vi "CookieGameEngine.vi"() -> (0 "PlayAgain":bool)   [LabVIEW 2020]
uses:
  typeDef/StateMachineEnum.ctl
  typeDef/EventData.ctl
  typeDef/EndType.ctl
  8a62bb5d-6283-479f-9ae8-d4a380ed6ac8.vi
panel:
  out "Picture":picture
  out "Time":string
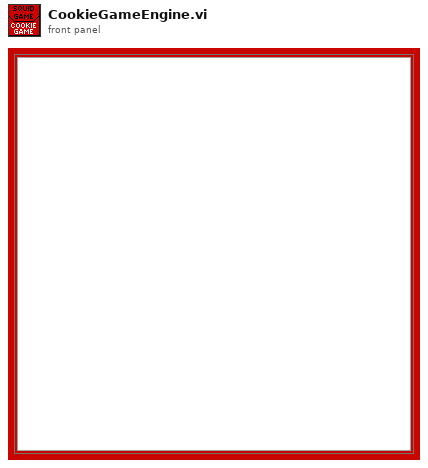
[diagram p1: front panel]
types:
  T1 = typedef "MainDataCluster.ctl" = cluster{"Image":T2, " TmpImage":T2, "BGColor":u32, "FGColor":u32, "DRColor":u32, "Picture":picture, "Queue ":refnum<queue>, "EndGameEvent":refnum<user-event>, "AnalizeMove":bool}
  T2 = typedef "imagedata.ctl" = cluster{"image type":i32, "image depth":i32, "image":u8[], "mask":u8[], "colors":u32[], "Rectangle":cluster{"left":i16, "top":i16, "right":i16, "bottom":i16}}
  T3 = typedef "StateMachineEnum.ctl" = enum16{"Init", "ReadTime", "StartTimer", "Result", "StopTimer", "ErrorHandler", "Close"}
  T4 = typedef "EventData.ctl" = cluster{"ShowResult":bool, "EndingType":T5}
  T5 = typedef "EndType.ctl" = enum16{"Timeout", "MouseUp", "OutOfLine", "CloseLine", "UserEnd"}
  T6 = typedef "LVMouseTypeDef.ctl" = cluster{"Mouse Position":cluster{"X":i32, "Y":i32}, "Mouse Modifiers":cluster{"Button Down":bool, "Shift Mod":bool, "Menu Mod":bool, "Option Mod":bool}}
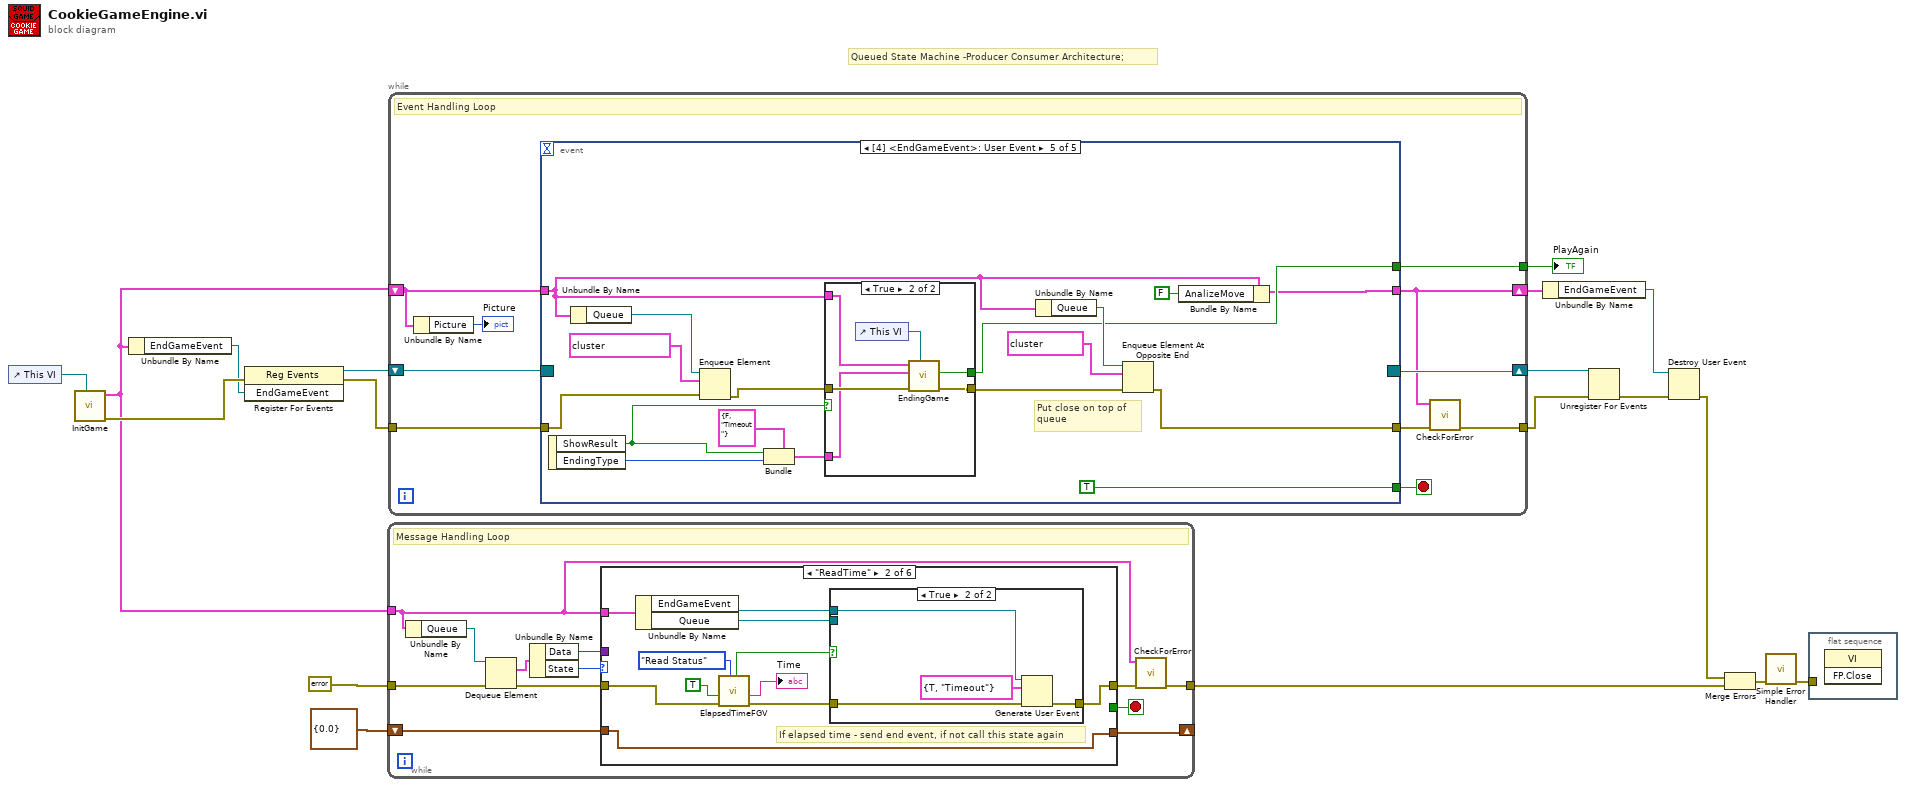
[diagram p0: block diagram]
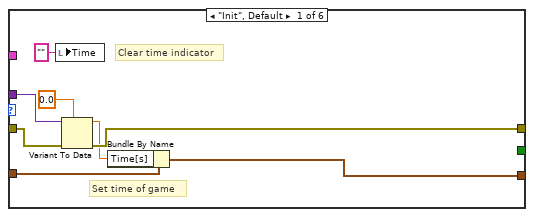
[diagram p2: hidden frame]
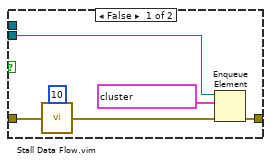
[diagram p3: hidden frame]
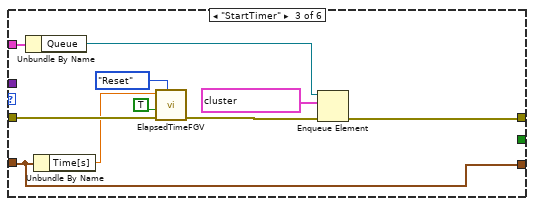
[diagram p4: hidden frame]
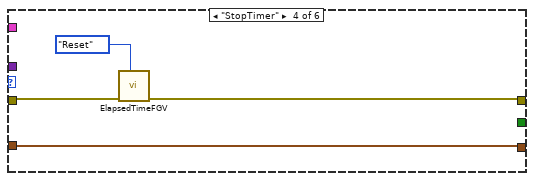
[diagram p5: hidden frame]
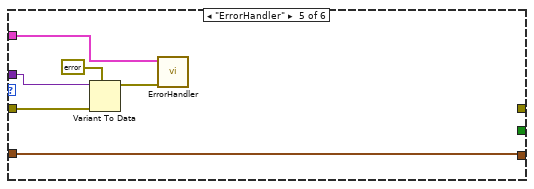
[diagram p6: hidden frame]
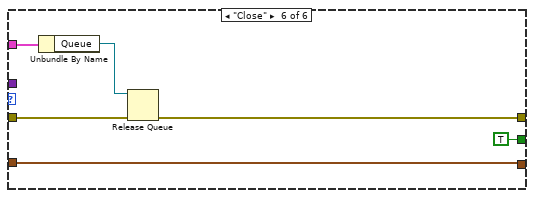
[diagram p7: hidden frame]
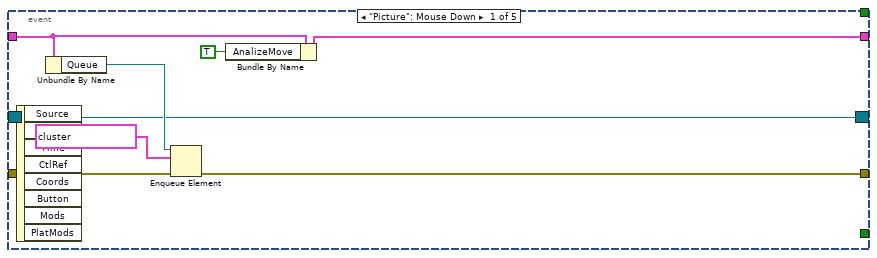
[diagram p8: hidden frame]
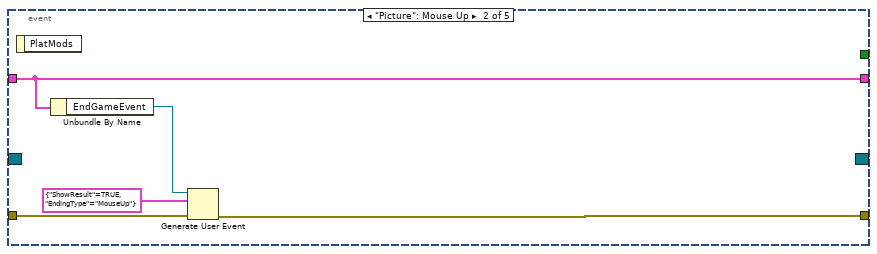
[diagram p9: hidden frame]
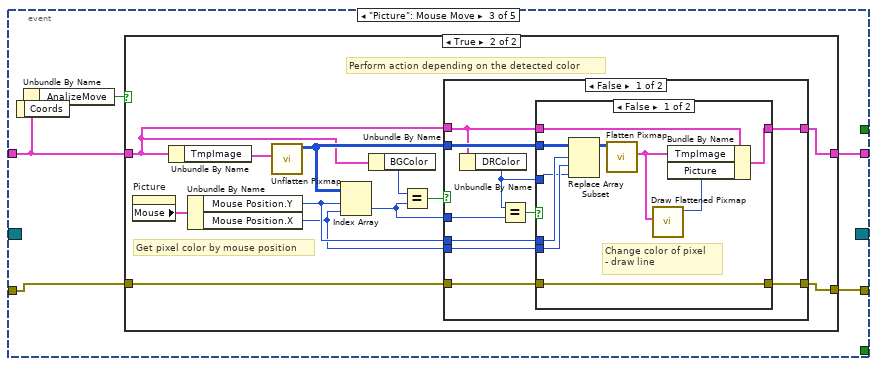
[diagram p10: hidden frame]
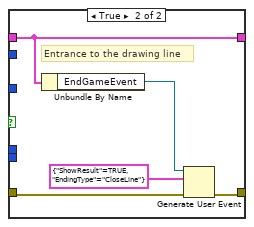
[diagram p12: hidden frame]
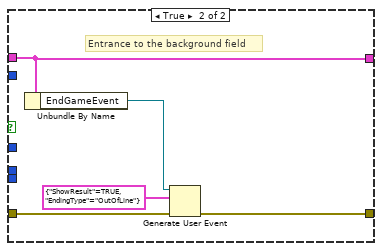
[diagram p13: hidden frame]
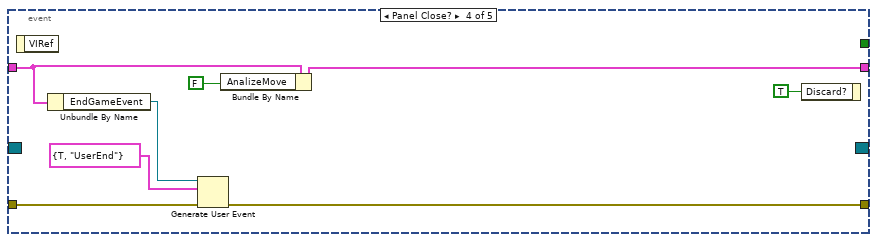
[diagram p14: hidden frame]
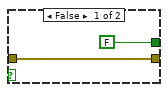
[diagram p15: hidden frame]
diagram:
  # "Queued State Machine -Producer Consumer Architecture;"
  n1 = control-ref of="This VI"() -> (w16:refnum<vi>)
  n2 = call "InitGame.vi"("VI Refnum"=w16) -> ("Error Out"=w14:errorcluster, "MainDataOut"=w10:T1)  [unwired: 9 in]
  n3 = Unbundle By Name(w10) -> ("EndGameEvent"=w1:refnum<user-event>)
  n4 = register-events(error in=w14, w1) -> (reference out=w2:refnum<event-registration>, error out=w13:errorcluster)  [unwired: 1 in]
  n5 = while {
    shift-right: [w23] -> _
    shift-left: cluster{"Time[s]":dbl} {"Time[s]"=0.0} -> [w24]
    tunnel: w10 -> [w19]
    tunnel: errorcluster {"status"=FALSE, "code"=0, "source"=""} ("error out") -> [w26]
    tunnel: [w20] -> w15
    stop <- w22 stop-if-true
    # "Message Handling Loop"
    n6 = Unbundle By Name(w19) -> ("Queue"=w21:refnum<queue>)
    n7 = Dequeue Element(queue=w21, error in (no error)=w26) -> (element=w30:cluster{"Data":variant, "State":T3}, error out=w28:errorcluster)  [unwired: 1 in, 2 out]
    n8 = Unbundle By Name(w30) -> ("Data"=w27:variant, "State"=w29:T3)
    n9 = case shown="\"ReadTime\"" w29 {
      tunnel: w28 -> [w37 w49 w68 w72 w78 w83]
      tunnel: w27 -> [w35 _ _ _ w79 _]
      tunnel: [w36 w47 w63 w71 _ w80] -> w25
      tunnel: w24 -> [w34 w46 w69 w73 w76 w84]
      tunnel: [w32 w46 w69 w73 w76 w84] -> w23
      tunnel: [_ _ _ _ _ TRUE] -> w22
      tunnel: w19 -> [_ w43 w61 _ w74 w82]
      frame "Init", Default {
        # "Clear time indicator"
        # "Set time of game"
        n10 = local write "Time"("" ("Time")) -> ()
        n11 = Variant To Data(error in=w37, type=0.0, Variant=w35) -> (data=w33:dbl, error out=w36:errorcluster)
        n12 = Bundle By Name(cluster=w34, "Time[s]"=w33) -> (w32:cluster{"Time[s]":dbl})
      }
      frame "ReadTime" {
        # "If elapsed time - send end event, if not call this state again"
        n13 = Unbundle By Name(w43) -> ("EndGameEvent"=w42:refnum<user-event>, "Queue"=w39:refnum<queue>)
        n14 = call "ElapsedTimeFGV.vi"("Timer  Mode"=enum16{"Reset", "Read Status", "Set Auto Reset"}."Read Status", "Error In"=w49, "Auto Reset (F)"=TRUE) -> ("Error Out"=w45:errorcluster, "Time left(s)"=→"Time":string, "Time Has Elapsed"=w44:bool)  [unwired: 5 in, 1 out]
        n15 = case shown="True" w44 {
          tunnel: w45 -> [w55 w59]
          tunnel: [w54 w58] -> w47
          tunnel: w42 -> [_ w57]
          tunnel: w39 -> [w52 _]
          frame False {
            n16 = call "Stall Data Flow.vim"("value in"=w55, "milliseconds to wait"=u32 10) -> ("value out"=w51:errorcluster)  [unwired: 1 out]
            n17 = Enqueue Element(queue=w52, element=cluster{"Data":variant, "State":T3} {"Data"=variant, "State"=enum."ReadTime"}, error in (no error)=w51) -> (error out=w54:errorcluster)  [unwired: 1 in, 2 out]
          }
          frame True {
            n18 = Generate User Event(user event=w57, event data cluster=T4 {"ShowResult"=TRUE, "EndingType"=enum."Timeout"} ("event data"), error in=w59) -> (error out=w58:errorcluster)  [unwired: 1 in, 1 out]
          }
        }
      }
      frame "StartTimer" {
        n19 = Unbundle By Name(w61) -> ("Queue"=w60:refnum<queue>)
        n20 = Unbundle By Name(w69) -> ("Time[s]"=w67:dbl)
        n21 = call "ElapsedTimeFGV.vi"("Timer  Mode"=enum16{"Reset", "Read Status", "Set Auto Reset"}."Reset", "Error In"=w68, "Auto Reset (F)"=TRUE, "Time Limit (s)"=w67) -> ("Error Out"=w64:errorcluster)  [unwired: 4 in, 3 out]
        n22 = Enqueue Element(queue=w60, element=cluster{"Data":variant, "State":T3} {"Data"=variant, "State"=enum."ReadTime"}, error in (no error)=w64) -> (error out=w63:errorcluster)  [unwired: 1 in, 2 out]
      }
      frame "StopTimer" {
        n23 = call "ElapsedTimeFGV.vi"("Timer  Mode"=enum16{"Reset", "Read Status", "Set Auto Reset"}."Reset", "Error In"=w72) -> ("Error Out"=w71:errorcluster)  [unwired: 6 in, 3 out]
      }
      frame "ErrorHandler" {
        n24 = Variant To Data(error in=w78, type=errorcluster {"status"=FALSE, "code"=0, "source"=""} ("error in (no error)"), Variant=w79) -> (data=w75:errorcluster)  [unwired: 1 out]
        n25 = call "ErrorHandler.vi"("Error In"=w75, "MainDataIn"=w74) -> ()  [unwired: 10 in]
      }
      frame "Close" {
        n26 = Unbundle By Name(w82) -> ("Queue"=w81:refnum<queue>)
        n27 = Release Queue(queue=w81, error in (no error)=w83) -> (error out=w80:errorcluster)  [unwired: 1 in, 2 out]
      }
    }
    n28 = call "CheckForError.vi"("Error In"=w25, "MainData In"=w19) -> ("Error Out"=w20:errorcluster)  [unwired: 9 in]
  }
  n29 = while {
    shift-right: [w86] -> w8
    shift-left: w10 -> [w91]
    tunnel: [w89] -> w12
    tunnel: w13 -> [w94]
    tunnel: [w87] -> w6
    shift-right: [w92] -> w3
    shift-left: w2 -> [w88]
    stop <- w95 stop-if-true
    # "Event Handling Loop"
    n30 = Unbundle By Name(w91) -> ("Picture"=→"Picture":picture)
    n31 = event shown="[4] <EndGameEvent>: User Event" {
      selector: w88 -> [w98 _ _ _ _]
      dyn-events: [w98 _ _ _ _] -> w92
      timeout: _ -> [_ _ _ _ _]
      tunnel: [_ _ _ _ TRUE] -> w95
      tunnel: w94 -> [w103 w108 w113 w165 w174]
      tunnel: [w102 w107 w110 w163 w180] -> w93
      tunnel: w91 -> [w101 w106 w112 w162 w170]
      tunnel: [w97 w106 w109 w159 w167] -> w86
      tunnel: [_ _ _ _ w175] -> w89
      event "Picture": Mouse Down {
        n32 = event-data() -> ()  [unwired: 1 in, 8 out]
        n33 = Unbundle By Name(w101) -> ("Queue"=w100:refnum<queue>)
        n34 = Enqueue Element(queue=w100, element=cluster{"Data":variant, "State":T3} {"Data"=variant, "State"=enum."StartTimer"}, error in (no error)=w103) -> (error out=w102:errorcluster)  [unwired: 1 in, 2 out]
        n35 = Bundle By Name(cluster=w101, "AnalizeMove"=TRUE) -> (w97:T1)
      }
      event "Picture": Mouse Up {
        n36 = event-data() -> ()  [unwired: 1 in, 1 out]
        n37 = Unbundle By Name(w106) -> ("EndGameEvent"=w105:refnum<user-event>)
        n38 = Generate User Event(user event=w105, event data cluster=T4 {"ShowResult"=TRUE, "EndingType"=enum."MouseUp"} ("event data"), error in=w108) -> (error out=w107:errorcluster)  [unwired: 1 in, 1 out]
      }
      event "Picture": Mouse Move {
        n39 = event-data() -> ()  [unwired: 1 in, 1 out]
        n40 = Unbundle By Name(w112) -> ("AnalizeMove"=w111:bool)
        n41 = case shown="True" w111 {
          tunnel: w112 -> [w115 w120]
          tunnel: w113 -> [w114 w119]
          tunnel: [w115 w117] -> w109
          tunnel: [w114 w116] -> w110
          frame False {
            # "Do nothing"
          }
          frame True {
            # "Perform action depending on the detected color"
            # "Get pixel color by mouse position"
            n42 = property on="Picture" class="Pict"() -> ("Mouse"=w118:T6)  [unwired: 2 in, 2 out]
            n43 = Unbundle By Name(w120) -> ("TmpImage"=w126:T2)
            n44 = Unbundle By Name(w118) -> ("Mouse Position.Y"=w122:i32, "Mouse Position.X"=w121:i32)
            n45 = call <vilib>:"Unflatten Pixmap.vi"("image data"=w126) -> ("24-bit pixmap"=w127:u32[][])  [unwired: 4 in, 6 out]
            n46 = Index Array(array=w127, index (row)=w122, index (col)=w121) -> (element=w125:u32)
            n47 = Unbundle By Name(w120) -> ("BGColor"=w123:u32)
            n48 = Equal?(x=w123, y=w125) -> (x = y?=w124:bool)
            n49 = case shown="False" w124 {
              tunnel: w127 -> [w137 _]
              tunnel: w122 -> [w136 _]
              tunnel: w121 -> [w135 _]
              tunnel: w125 -> [w133 _]
              tunnel: [w132 w155] -> w116
              tunnel: w120 -> [w131 w157]
              tunnel: [w129 w157] -> w117
              tunnel: w119 -> [w128 w156]
              frame False {
                n50 = Unbundle By Name(w131) -> ("DRColor"=w130:u32)
                n51 = Equal?(x=w130, y=w133) -> (x = y?=w134:bool)
                n52 = case shown="False" w134 {
                  tunnel: w137 -> [w147 _]
                  tunnel: w136 -> [w146 _]
                  tunnel: w135 -> [w145 _]
                  tunnel: [w138 w151] -> w132
                  tunnel: w131 -> [w142 w150]
                  tunnel: w130 -> [w143 _]
                  tunnel: [w139 w150] -> w129
                  tunnel: w128 -> [w138 w152]
                  frame False {
                    # "Change color of pixel \n- draw line"
                    n53 = Replace Array Subset(array=w147, new element=w143, index (row)=w146, index (col)=w145) -> (w144:u32[][])
                    n54 = call <vilib>:"Flatten Pixmap.vi"("24-bit pixmap"=w144) -> ("image data"=w141:T2)  [unwired: 10 in]
                    n55 = call <vilib>:"Draw Flattened Pixmap.vi"("image data"=w141) -> ("new picture"=w140:picture)  [unwired: 8 in]
                    n56 = Bundle By Name(cluster=w142, "TmpImage"=w141, "Picture"=w140) -> (w139:T1)
                  }
                  frame True {
                    # "Entrance to the drawing line"
                    n57 = Unbundle By Name(w150) -> ("EndGameEvent"=w149:refnum<user-event>)
                    n58 = Generate User Event(user event=w149, event data cluster=T4 {"ShowResult"=TRUE, "EndingType"=enum."CloseLine"} ("event data"), error in=w152) -> (error out=w151:errorcluster)  [unwired: 1 in, 1 out]
                  }
                }
              }
              frame True {
                # "Entrance to the background field"
                n59 = Unbundle By Name(w157) -> ("EndGameEvent"=w154:refnum<user-event>)
                n60 = Generate User Event(user event=w154, event data cluster=T4 {"ShowResult"=TRUE, "EndingType"=enum."OutOfLine"} ("event data"), error in=w156) -> (error out=w155:errorcluster)  [unwired: 1 in, 1 out]
              }
            }
          }
        }
      }
      event Panel Close? {
        n61 = event-data() -> ()  [unwired: 1 in, 1 out]
        n62 = Unbundle By Name(w162) -> ("EndGameEvent"=w161:refnum<user-event>)
        n63 = Generate User Event(user event=w161, event data cluster=T4 {"ShowResult"=TRUE, "EndingType"=enum."UserEnd"} ("event data"), error in=w165) -> (error out=w163:errorcluster)  [unwired: 1 in, 1 out]
        n64 = Bundle By Name(cluster=w162, "AnalizeMove"=FALSE) -> (w159:T1)
        n65 = event-data("Discard?"=TRUE) -> ()  [unwired: 1 in, 1 out]
      }
      event User Event {
        # "Put close on top of \nqueue"
        n66 = event-data() -> ("ShowResult"=w168:bool, "EndingType"=w173:T5)  [unwired: 1 in]
        n67 = Unbundle By Name(w170) -> ("Queue"=w179:refnum<queue>)
        n68 = Enqueue Element(queue=w179, element=cluster{"Data":variant, "State":T3} {"Data"=variant, "State"=enum."StopTimer"}, error in (no error)=w174) -> (error out=w181:errorcluster)  [unwired: 1 in, 2 out]
        n69 = Bundle(cluster=T4 {"ShowResult"=FALSE, "EndingType"=enum."Timeout"} ("EndData"), "ShowResult"=w168, "EndingType"=w173) -> (w169:T4)
        n70 = case shown="True" w168 {
          tunnel: [w183 w189] -> w182
          tunnel: w181 -> [w183 w188]
          tunnel: [FALSE ("PlayAgain") w187] -> w175
          tunnel: w169 -> [_ w186]
          tunnel: w170 -> [_ w185]
          frame False {
          }
          frame True {
            n71 = control-ref of="This VI"() -> (w190:refnum<vi>)
            n72 = call "EndingGame.vi"("VI Refnum"=w190, "Error In"=w188, "EndData"=w186, "MainData"=w185) -> ("Error Out"=w189:errorcluster, "PlayAgain"=w187:bool)  [unwired: 6 in]
          }
        }
        n73 = Unbundle By Name(w170) -> ("Queue"=w178:refnum<queue>)
        n74 = Enqueue Element At Opposite End(queue=w178, element=cluster{"Data":variant, "State":T3} {"Data"=variant, "State"=enum."Close"}, error in (no error)=w182) -> (error out=w180:errorcluster)  [unwired: 1 in, 2 out]
        n75 = Bundle By Name(cluster=w170, "AnalizeMove"=FALSE) -> (w167:T1)
      }
    }
    n76 = call "CheckForError.vi"("Error In"=w93, "MainData In"=w86) -> ("Error Out"=w87:errorcluster)  [unwired: 9 in]
  }
  "PlayAgain" <- w12
  n77 = Unbundle By Name(w8) -> ("EndGameEvent"=w7:refnum<user-event>)
  n78 = Unregister For Events(event registration refnum=w3, error in=w6) -> (error out=w9:errorcluster)
  n79 = Destroy User Event(user event=w7, error in=w9) -> (error out=w5:errorcluster)
  n80 = Merge Errors(w5, w15) -> (w11:errorcluster)
  n81 = call <vilib>:"Simple Error Handler.vi"("error in (no error)"=w11) -> ("error out"=w4:errorcluster)  [unwired: 4 in, 4 out]
  n82 = flat-sequence {
    tunnel: w4 -> [_]
    frame #0 {
      n83 = invoke class="VI" method="FP.Close"() -> ()  [unwired: 3 in, 3 out]
    }
  }
